vi "Read Restarted Flag.vi"(8 "error in (no error)":errorcluster, 11 "PLBB in":refnum<class "PL BlackBox Modbus Client.lvclass">) -> (0 "error out":errorcluster, 2 "restarted flag":bool, 3 "PLBB out":refnum<class "PL BlackBox Modbus Client.lvclass">)   [LabVIEW 2015, in "PL BlackBox Modbus Client.lvclass"]
doc: "Reads the restarted flag."
uses:
  PL BlackBox Modbus Client.lvclass
  <vilib>/plasmapper/PL Modbus Client/PL Modbus Client.lvclass
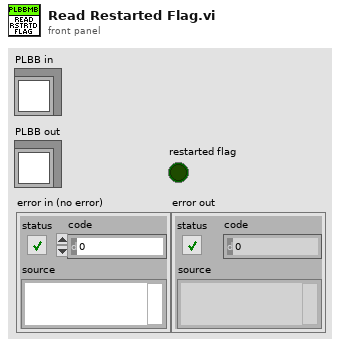
[diagram p1: front panel]
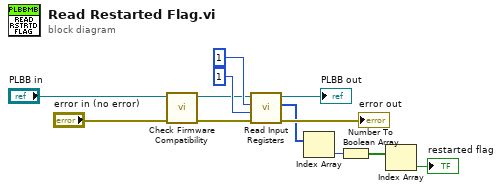
[diagram p0: block diagram]
diagram:
  n1 = call-dynamic "Check Firmware Compatibility.vi"("error in (no error)"="error in (no error)", "PLBB in"="PLBB in") -> ("error out"=w6:errorcluster, "PLBB out"=w5:refnum<class "PL BlackBox Modbus Client.lvclass">)  [unwired: 8 in]
  n2 = call <vilib>:"Read Input Registers.vi"("error in (no error)"=w6, "number of input registers"=u16 1 ("address"), "address"=u16 1, "MODBUS in"=w5) -> ("error out"=→"error out":errorcluster, "values"=w4:u16[], "MODBUS out"=→"PLBB out":refnum<class "PL BlackBox Modbus Client.lvclass">)  [unwired: 5 in]
  n3 = Index Array(array=w4) -> (element=w3:u16)  [unwired: 1 in]
  n4 = Number To Boolean Array(number=w3) -> (Boolean array=w2:bool[])
  n5 = Index Array(array=w2) -> (element=→"restarted flag":bool)  [unwired: 1 in]
